vi "CREATE_COMMANDS_FOR_LAKESHORE.vi"(10 "Channel":string, 11 "Select Parameter":enum16{"Resistance(ohms)", "Temperature(K)"}(ring)) -> (3 "result string":string)   [LabVIEW 2020]
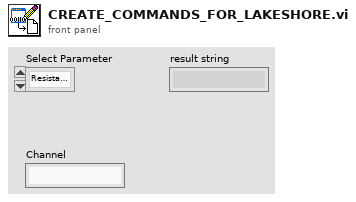
[diagram p1: front panel]
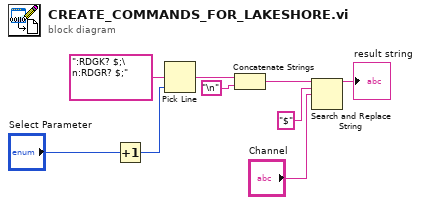
[diagram p0: block diagram]
diagram:
  n1 = Increment(x="Select Parameter") -> (x+1=w6:enum16{"Resistance(ohms)", "Temperature(K)"})
  n2 = Pick Line(multi-line string=":RDGK? $;\n:RDGR? $;", line index=w6) -> (output string=w7:string)  [unwired: 1 in]
  n3 = Concatenate Strings(w7, "\n") -> (w9:string)
  n4 = Search and Replace String(input string=w9, search string="$", replace string="Channel") -> (result string=→"result string":string)  [unwired: 5 in, 3 out]
